vi "fill in.vi"   [LabVIEW 2023]
types:
  T1 = enum16{"plate1", "plate2", "plate3", "rinse", "seat"}
  T2 = enum16{"Initialize", "Absolute Position", "Relative Pickup", "Relative Dispense", "Swich valve", "Bypass"}
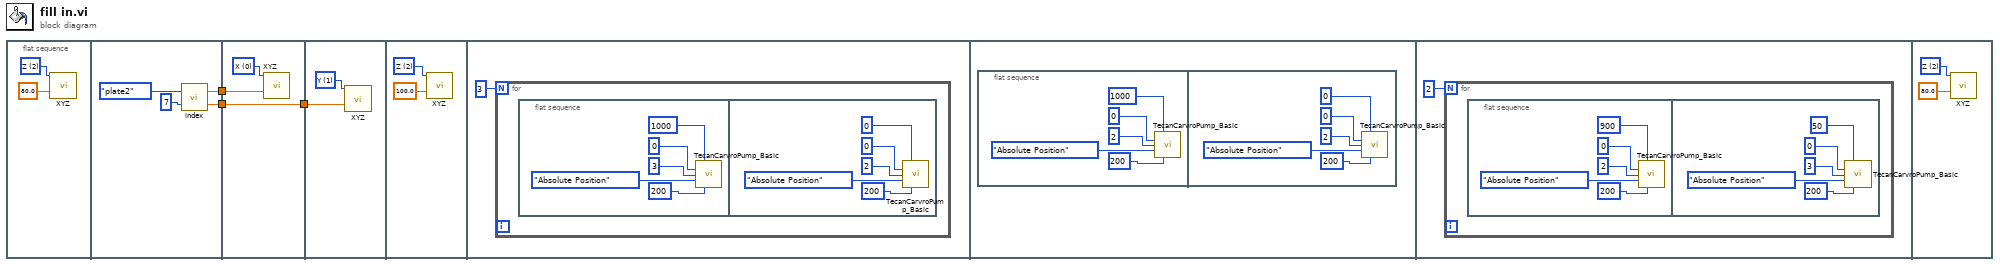
[diagram p0: block diagram]
diagram:
  n1 = flat-sequence {
    tunnel: [w9] -> w3
    tunnel: [w8] -> w2
    tunnel: w3 -> [w12]
    tunnel: [w10] -> w1
    tunnel: w2 -> [w10]
    tunnel: w1 -> [w13]
    frame #0 {
      w5 = u16 2 items=["X", "Y", "Z"] ("AXIS")
      n2 = call "XYZ.vi"("AXIS"=w5, "Set location (mm)"=80.0) -> ()  [unwired: 9 in, 5 out]
    }
    frame #1 {
      n3 = call "index.vi"("index"=i8 7, "where"=T1."plate2") -> ("Y"=w8:dbl, "X"=w9:dbl)
    }
    frame #2 {
      w11 = u16 0 items=["X", "Y", "Z"] ("AXIS")
      n4 = call "XYZ.vi"("AXIS"=w11, "Set location (mm)"=w12) -> ()  [unwired: 9 in, 5 out]
    }
    frame #3 {
      w14 = u16 1 items=["X", "Y", "Z"] ("AXIS")
      n5 = call "XYZ.vi"("AXIS"=w14, "Set location (mm)"=w13) -> ()  [unwired: 9 in, 5 out]
    }
    frame #4 {
      w16 = u16 2 items=["X", "Y", "Z"] ("AXIS")
      n6 = call "XYZ.vi"("AXIS"=w16, "Set location (mm)"=100.0) -> ()  [unwired: 9 in, 5 out]
    }
    frame #5 {
      n7 = for {
        N: 3 -> [_]
        n8 = flat-sequence {
          frame #0 {
            n9 = call "TecanCarvroPump_Basic.vi"("Volume (μL)"=u16 1000, "TecanPump address"=u8 0, "Valve"=u8 3, "Mode"=T2."Absolute Position", "Speed (μL/s)"=u16 200) -> ()  [unwired: 10 in, 1 out]
          }
          frame #1 {
            n10 = call "TecanCarvroPump_Basic.vi"("Volume (μL)"=u16 0, "TecanPump address"=u8 0, "Valve"=u8 2, "Mode"=T2."Absolute Position", "Speed (μL/s)"=u16 200) -> ()  [unwired: 10 in, 1 out]
          }
        }
      }
    }
    frame #6 {
      n11 = flat-sequence {
        frame #0 {
          n12 = call "TecanCarvroPump_Basic.vi"("Volume (μL)"=u16 1000, "TecanPump address"=u8 0, "Valve"=u8 2, "Mode"=T2."Absolute Position", "Speed (μL/s)"=u16 200) -> ()  [unwired: 10 in, 1 out]
        }
        frame #1 {
          n13 = call "TecanCarvroPump_Basic.vi"("Volume (μL)"=u16 0, "TecanPump address"=u8 0, "Valve"=u8 2, "Mode"=T2."Absolute Position", "Speed (μL/s)"=u16 200) -> ()  [unwired: 10 in, 1 out]
        }
      }
    }
    frame #7 {
      n14 = for {
        N: 2 -> [_]
        n15 = flat-sequence {
          frame #0 {
            n16 = call "TecanCarvroPump_Basic.vi"("Volume (μL)"=u16 900, "TecanPump address"=u8 0, "Valve"=u8 2, "Mode"=T2."Absolute Position", "Speed (μL/s)"=u16 200) -> ()  [unwired: 10 in, 1 out]
          }
          frame #1 {
            n17 = call "TecanCarvroPump_Basic.vi"("Volume (μL)"=u16 50, "TecanPump address"=u8 0, "Valve"=u8 3, "Mode"=T2."Absolute Position", "Speed (μL/s)"=u16 200) -> ()  [unwired: 10 in, 1 out]
          }
        }
      }
    }
    frame #8 {
      w50 = u16 2 items=["X", "Y", "Z"] ("AXIS")
      n18 = call "XYZ.vi"("AXIS"=w50, "Set location (mm)"=80.0) -> ()  [unwired: 9 in, 5 out]
    }
  }
